vi "fill_in_missing_pressures.vi"(10 "Default Pressures":dbl[](array[numeric])=[301.07330322265625, 823.0598754882812, 366.0849609375, 327.5828857421875], 11 "Pressure Sequence":dbl[][](array[numeric])) -> (3 "Pressure Sequence Out":dbl[][](array[numeric]))   [LabVIEW 2016]
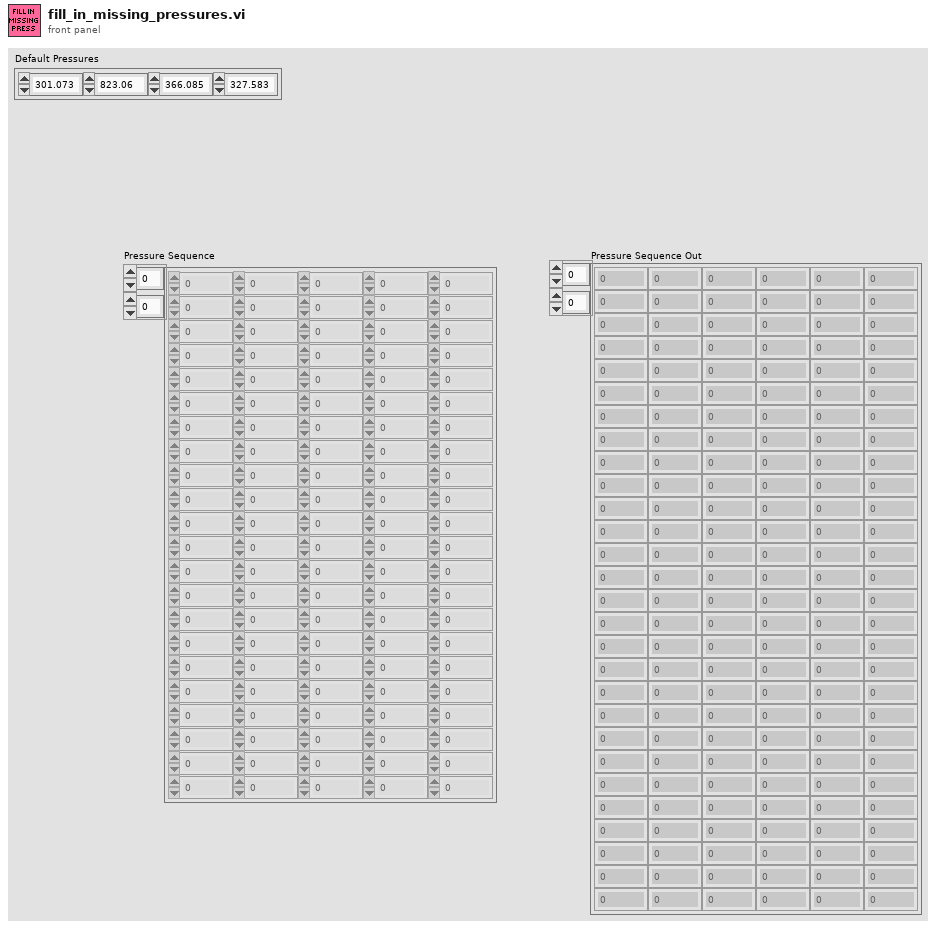
[diagram p1: front panel]
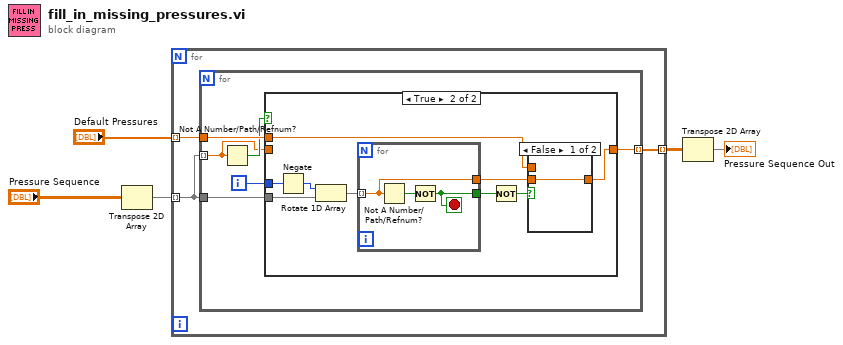
[diagram p0: block diagram]
diagram:
  n1 = Transpose 2D Array(2D array="Pressure Sequence") -> (transposed array=w2:dbl[][])
  n2 = for {
    tunnel: w2 -> [w6] mode=indexing
    tunnel: "Default Pressures" -> [w8] mode=indexing
    tunnel: [w7] -> w3 mode=indexing
    n3 = for {
      tunnel: w6 -> [w9] mode=indexing
      tunnel: w8 -> [w14]
      tunnel: [w13] -> w7 mode=indexing
      tunnel: w6 -> [w11]
      i -> [w12]
      n4 = Not A Number/Path/Refnum?(number/path/refnum=w9) -> (NaN/Path/Refnum?=w10:bool)
      n5 = case shown="True" w10 {
        tunnel: w14 -> [_ w24]
        tunnel: [w15 w23] -> w13
        tunnel: w12 -> [_ w20]
        tunnel: w11 -> [_ w21]
        tunnel: w9 -> [w15 _]
        frame False {
        }
        frame True {
          n6 = Negate(x=w20) -> (-x=w18:i32)
          n7 = Rotate 1D Array(1:w21, 2:w18) -> (0:w19:dbl[])
          n8 = for {
            tunnel: w19 -> [w27] mode=indexing
            tunnel: [w27] -> w16
            tunnel: [w25] -> w22
            stop <- w25 stop-if-true
            n9 = Not A Number/Path/Refnum?(number/path/refnum=w27) -> (NaN/Path/Refnum?=w26:bool)
            n10 = Not(x=w26) -> (.not. x?=w25:bool)
          }
          n11 = Not(x=w22) -> (.not. x?=w17:bool)
          n12 = case shown="False" w17 {
            tunnel: [w28 w29] -> w23
            tunnel: w24 -> [_ w29]
            tunnel: w16 -> [w28 _]
            frame False {
            }
            frame True {
            }
          }
        }
      }
    }
  }
  n13 = Transpose 2D Array(2D array=w3) -> (transposed array=→"Pressure Sequence Out":dbl[][])
